vi "Configure Master.vi"(8 "error in":errorcluster, 10 "Cyclic Data Bandwidth":u32, 11 "IOV ref in":refnum<k21>) -> (0 "error out":errorcluster, 2 "Cyclic Data Bandwidth out":u32, 3 "IOV ref out":refnum<k21>)   [LabVIEW 2016, in "Scan Engine Custom Device.lvlib"]
uses:
  Scan Engine Custom Device.lvlib
  <resource>/objmgr/IndComECAT.rc
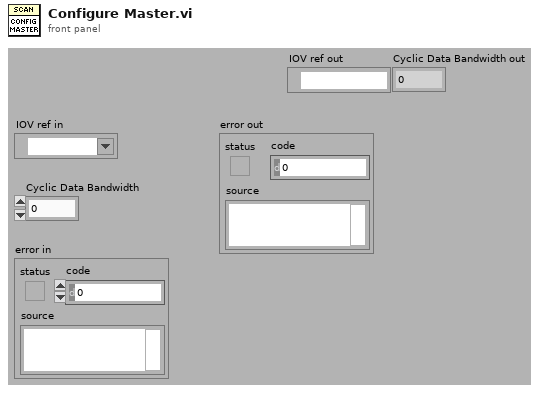
[diagram p1: front panel]
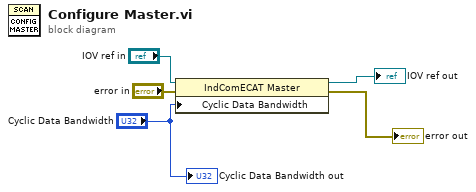
[diagram p0: block diagram]
diagram:
  n1 = property class="IndComECAT Master"(reference="IOV ref in", error in="error in", "Cyclic Data Bandwidth"="Cyclic Data Bandwidth") -> (reference out=→"IOV ref out":refnum<k21>, error out=→"error out":errorcluster)
  "Cyclic Data Bandwidth out" <- "Cyclic Data Bandwidth"
